vi "Set Fail Code.vi"(8 "error in (no error)":errorcluster, 10 "Fail Code":string, 11 "Test Class in":refnum<class "Test Class.lvclass">) -> (0 "error out":errorcluster, 3 "Test Class out":refnum<class "Test Class.lvclass">)   [LabVIEW 2015, in "Test Class.lvclass"]
uses:
  Test Class.lvclass
  Test Class.lvclass/Test Class.ctl
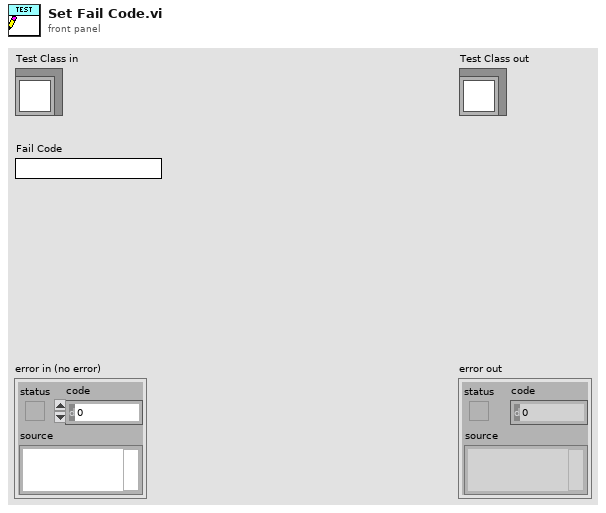
[diagram p1: front panel]
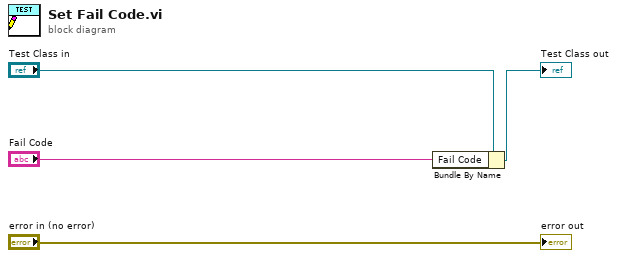
[diagram p0: block diagram]
diagram:
  n1 = Bundle By Name(cluster="Test Class in", "Fail Code"="Fail Code") -> (→"Test Class out":refnum<class "Test Class.lvclass">)
  "error out" <- "error in (no error)"
